vi "PH_Beckhoff_StepMot.set Axis Settings to GUI.vi"(0 "VI in":refnum<vi>, 5 "error in (no error)":errorcluster) -> (14 "VI out":refnum<vi>, 19 "error out":errorcluster)   [LabVIEW 2014, in "PH_Beckhoff_StepMot.lvlib"]
uses:
  PH_Beckhoff_StepMot.lvlib
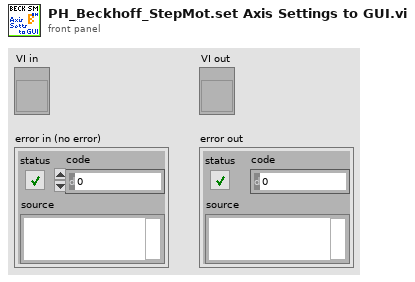
[diagram p1: front panel]
types:
  T1 = typedef "PH_Beckhoff_StepMot.lvlib/PH_Beckhoff_StepMot.i attribute.ctl" = cluster{"Axes Settings":T2[], "GUI Refs":cluster{"Axes Settings":refnum<vi>, "Stati":refnum<vi>}, "Get Beckhoff Settings":bool}
  T2 = typedef "PH_Beckhoff_StepMot.lvlib/PH_Beckhoff_StepMot.Axis Cluster.ctl" = cluster{"Step Motor Configuration":T3, "To set?":bool, "Endswitch inverted?":bool}
  T3 = typedef "Beckhoff - Driver np.lvlib/Beckhoff.Step Motor - Motor Configuration.ctl" = cluster{"Feature Register":T4, "I max A [mA]":dbl, "I max B [mA]":dbl, "v min":u32, "v max":u32, "a max":u32, "I hold [%]":u32, "Steps/qp":u32, "Feature Register 2":T5}
  T4 = typedef "Beckhoff - Driver np.lvlib/Beckhoff.Step Motor - Feature Register 1.ctl" = cluster{"en Auto Start":bool, "en Auto Stop":bool, "dis Wd Timer":bool, "OP Mode 1":bool, "OP Mode 2":bool, "Ramp Type":bool, "inv Pos Feedback":bool, "en User Cur Table":bool, "en Latch Evt Clr Pos":bool, "en Multi Latch Vals":bool, "en Sign Disp*":bool, "Feedback Type*":bool, "en neg Gate Lock*":bool, "en pos Gate Lock*":bool, "dis Enc Fltr*":bool, "en Counter Mode*":bool}
  T5 = typedef "Beckhoff - Driver np.lvlib/Beckhoff.Step Motor - Feature Register 2.ctl" = cluster{"rev Homing Dir":bool, "en Decac Ramp":bool, "Latch Reg Pos":bool, "Show Idle":bool, "dis Ref Input 1":bool, "dis Ref Input 2":bool, "en ext Auto Start":bool, "N/A":bool, "N/A":bool, "N/A":bool, "N/A":bool, "N/A":bool, "en Clr Proc Data":bool, "en Man Ecl Tolerce*":bool, "rev Dig Input 1":bool, "rev Dig Input 2":bool}
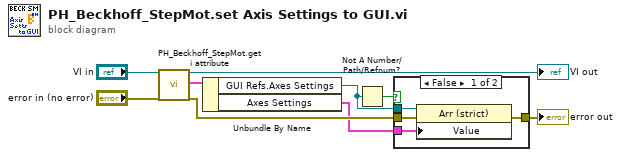
[diagram p0: block diagram]
diagram:
  n1 = call "PH_Beckhoff_StepMot.get i attribute.vi"("i ref in"="VI in", "error in (no error)"="error in (no error)") -> ("i ref out"=→"VI out":refnum<vi>, "i attribute"=w5:T1, "error out"=w9:errorcluster)  [unwired: 15 in]
  n2 = Unbundle By Name(w5) -> ("GUI Refs.Axes Settings"=w1:refnum<vi>, "Axes Settings"=w3:T2[])
  n3 = Not A Number/Path/Refnum?(number/path/refnum=w1) -> (NaN/Path/Refnum?=w2:bool)
  n4 = case shown="False" w2 {
    tunnel: w9 -> [w13 w14]
    tunnel: [w12 w14] -> w4
    tunnel: w1 -> [w11 _]
    tunnel: w3 -> [w10 _]
    frame False {
      n5 = property class="Arr (strict)"(reference=w11, error in=w13, "Value"=w10) -> (error out=w12:errorcluster)  [unwired: 1 out]
    }
    frame True {
    }
  }
  "error out" <- w4
